vi "Check for Errors.vi"(8 "error in":errorcluster, 11 "Engine in":refnum<class "Engine.lvclass">) -> (0 "error out":errorcluster, 3 "Engine out":refnum<class "Engine.lvclass">)   [LabVIEW 2019, in "Engine.lvlib" / "Engine.lvclass"]
doc: "This routine checks incoming error terminals and relays an error event to the fault handler if there is an error, removing the error from the terminal and allowing the software to continue executing\n\n*This VI will allow the error to pass through if the original error event was not created."
uses:
  Project/Engine.lvclass
  Project/Engine.lvclass/Engine.ctl
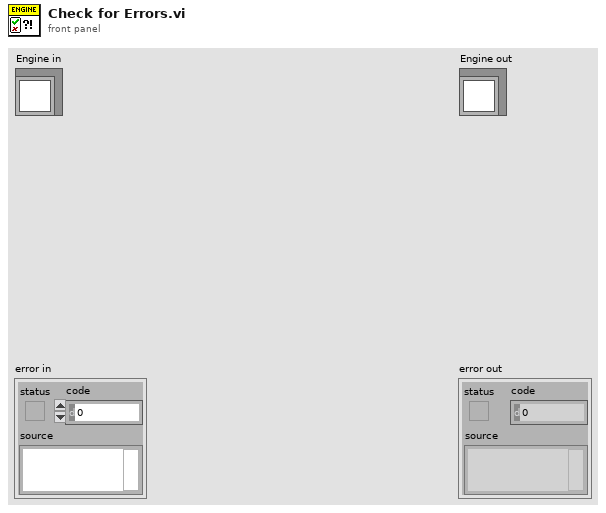
[diagram p1: front panel]
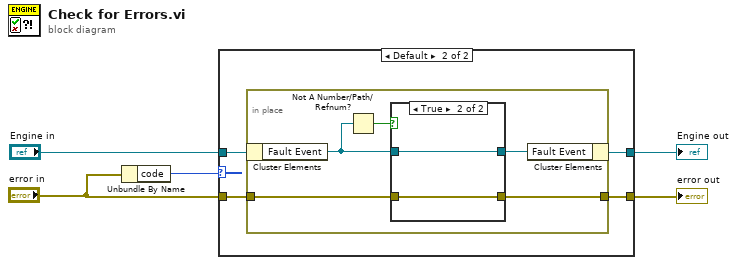
[diagram p0: block diagram]
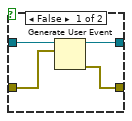
[diagram p3: hidden frame]
diagram:
  n1 = Unbundle By Name("error in") -> ("code"=w3:i32)
  n2 = case shown="Default" w3 {
    tunnel: "Engine in" -> [w7 w11]
    tunnel: [w7 w10] -> w4
    tunnel: "error in" -> [w6 w9]
    tunnel: [w6 w8] -> w1
    frame 0 {
    }
    frame Default {
      n3 = in-place {
        in-place-border: w9 -> [w15]
        in-place-border: [w14] -> w8
        n4 = in-place-cluster #1(w11) -> ("Fault Event"=w13:refnum<user-event>)
        n5 = Not A Number/Path/Refnum?(number/path/refnum=w13) -> (NaN/Path/Refnum?=w12:bool)
        n6 = case shown="True" w12 {
          tunnel: [w20 w22] -> w16
          tunnel: w15 -> [w19 w21]
          tunnel: [w18 w21] -> w14
          tunnel: w13 -> [w17 w22]
          frame False {
            n7 = Generate User Event(user event=w17, event data cluster=w19) -> (user event out=w20:refnum<user-event>, error out=w18:errorcluster)  [unwired: 2 in]
          }
          frame True {
          }
        }
        n8 = in-place-cluster #1("Fault Event"=w16) -> (w10:refnum<class "Engine.lvclass">)
      }
    }
  }
  "error out" <- w1
  "Engine out" <- w4
